vi "Init Camera.vi"(8 "error in (no error)":errorcluster, 10 "Physical Camera Assignment":T1[](array[typedef]), 11 "Photometrics Camera in":refnum<class "Photometrics Camera.lvclass">) -> (0 "error out":errorcluster, 3 "Photometrics Camera out":refnum<class "Photometrics Camera.lvclass">)   [LabVIEW 2022 SP3, in "Photometrics Camera.lvlib" / "Photometrics Camera.lvclass"]
uses:
  Photometrics Camera.lvclass
  Resources/Type Defs/Physical Camera Assignment.ctl
  Photometrics Camera.lvclass/Photometrics Camera.ctl
  Resources/GLOBAL/GLOBAL Time-critical.vi
  C:/FlashGordon/Development/dll/PVCamNET.dll
  dll/PVCamNET.dll
  Camera/Camera.lvclass
  Photometrics Camera.lvlib
panel:
  out "Selected Cameras":T1[](array[typedef])
  out "Version":string
  out "PVCamVersion":string
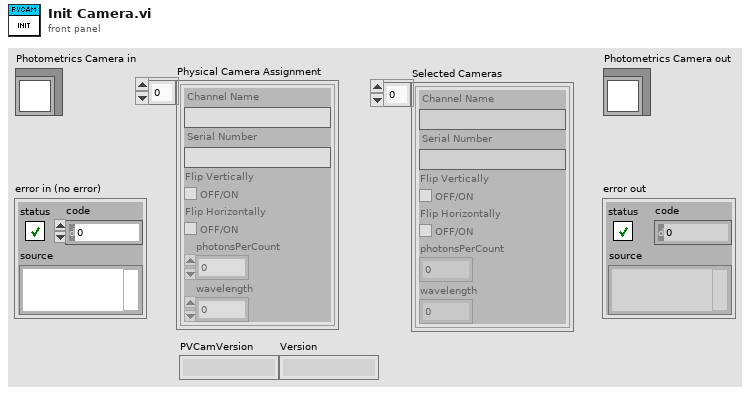
[diagram p1: front panel]
types:
  T1 = typedef "Physical Camera Assignment.ctl" = cluster{"Channel Name":string, "Serial Number":string, "Flip Vertically":bool, "Flip Horizontally":bool, "photonsPerCount":dbl, "wavelength":i16}
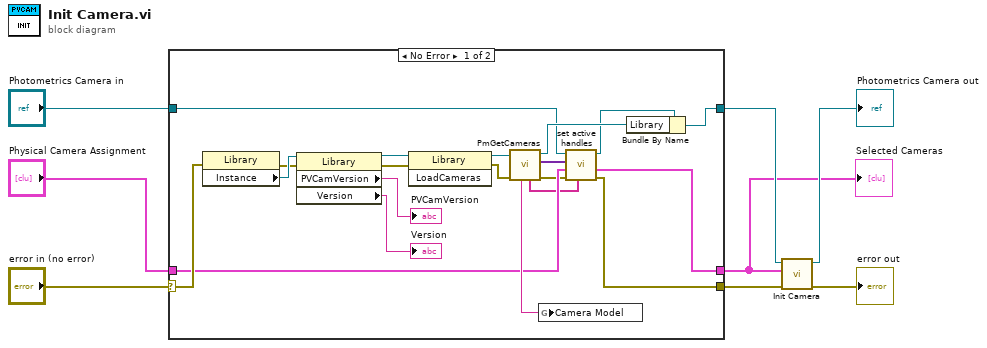
[diagram p0: block diagram]
diagram:
  n1 = case shown="No Error" "error in (no error)" {
    selector: "error in (no error)" -> [w17 w31]
    tunnel: [w11 w31] -> w6
    tunnel: [w18 w30] -> w4
    tunnel: "Photometrics Camera in" -> [w13 w30]
    tunnel: "Physical Camera Assignment" -> [w16 w29]
    tunnel: [w10 w29] -> w1
    frame No Error {
      n2 = property class="Library"(error in=w17) -> (error out=w25:errorcluster, "Instance"=w26:refnum<k24>)  [unwired: 1 in, 1 out]
      n3 = property class="Library"(reference=w26, error in=w25) -> (reference out=w23:refnum<k24>, error out=w24:errorcluster, "PVCamVersion"=→"PVCamVersion":string, "Version"=→"Version":string)
      n4 = invoke class="Library" method="LoadCameras"(reference=w23, error in=w24) -> (reference out=w28:refnum<k24>, error out=w27:errorcluster)  [unwired: 1 in, 1 out]
      n5 = call "PmGetCameras.vi"("error in (no error)"=w27, "Library"=w28) -> ("error out"=w14:errorcluster, "Cameras"=w9:variant[], "Library 2"=w19:refnum<k24>, "SN"=w15:string[], "Model"=w20:string)  [unwired: 5 in]
      n6 = global write "GLOBAL Time-critical.vi" "Camera Model"(w20) -> ()
      n7 = call-dynamic "set active handles.vi"("serial numbers"=w15, "error in (no error)"=w14, "All Camera"=w16, "All Handles"=w9, "Camera in"=w13) -> ("error out"=w11:errorcluster, "Selected cameras"=w10:T1[], "Camera out"=w12:refnum<class "Photometrics Camera.lvclass">)  [unwired: 3 in, 1 out]
      n8 = Bundle By Name(cluster=w12, "Library"=w19) -> (w18:refnum<class "Photometrics Camera.lvclass">)
    }
    frame Error {
    }
  }
  "Selected Cameras" <- w1
  n9 = call-parent "Init Camera.vi"("error in (no error)"=w6, "Physical Camera Assignment"=w1, "Camera in"=w4) -> ("error out"=→"error out":errorcluster, "Camera out"=→"Photometrics Camera out":refnum<class "Photometrics Camera.lvclass">)  [unwired: 7 in]
